vi "Draw Highlighted Tree rows.vi"(8 "error in (no error)":errorcluster, 9 "DragOver Output":T2={"Displayed Row"=0, "Position"=enum."On Row", "Row's TreeItem index"=0, "indent"=0, "Accepted?"=FALSE, "Insertion index"=0, "Top left visible TreeItem index"=0, "Bar type"=enum."tilda up"}, 10 "TreeItems":T1[](array[typedef]), 11 "TreeRef":refnum<vi>) -> (0 "error out":errorcluster)   [LabVIEW 2020, in "BetterDragAndDrop.lvlib" / "BetterTreeHandle.lvclass"]
uses:
  Classes/BetterTreeHandle/BetterTreeHandle.lvclass
  DragOver Output.ctl
  DragOverPosition.ctl
  Classes/BetterTreeBar/SubVIs/Horizontal Bar Enumeration.ctl
  Classes/BetterTreeItem/SubVIs/TreeItem.ctl
  Classes/BetterHandle/BetterHandle.lvclass
  Classes/BetterTreeBar/BetterHorizontalBar.lvclass
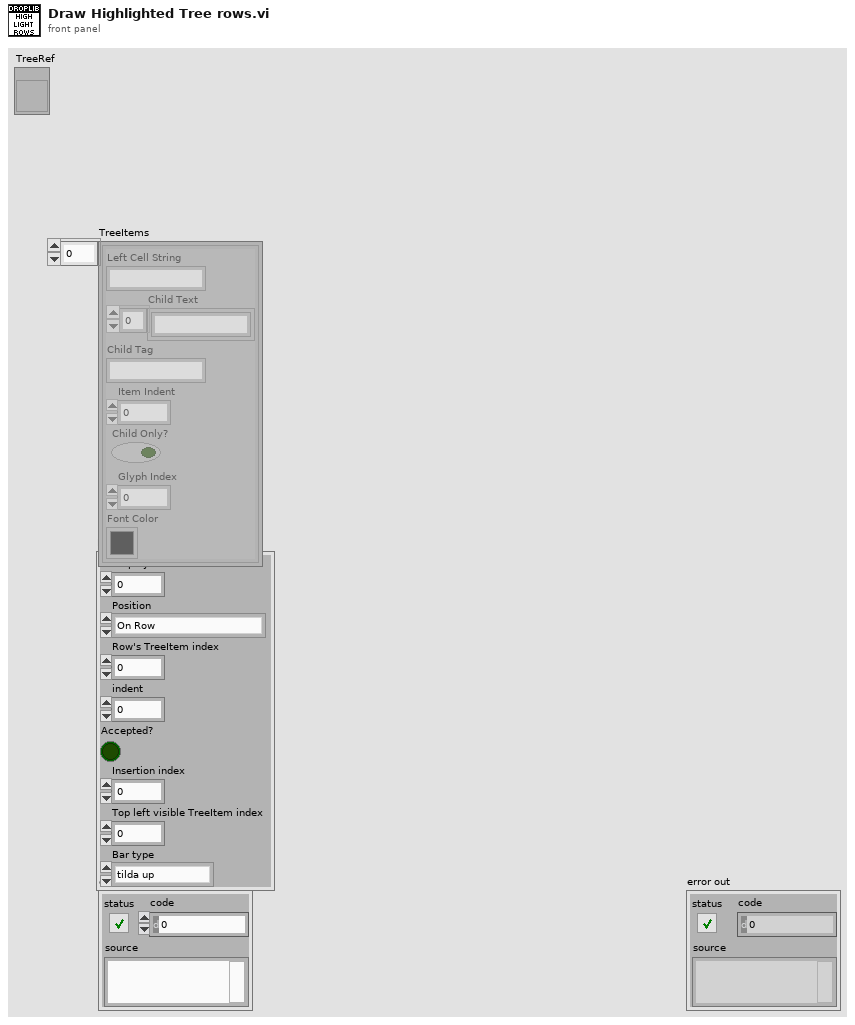
[diagram p1: front panel]
types:
  T1 = typedef "BetterDragAndDrop.lvlib/BetterTreeHandle.lvclass/TreeItem.ctl" = cluster{"Left Cell String":string, "Child Text":string[], "Child Tag":string, "Item Indent":i32, "Child Only?":bool, "Glyph Index":i32, "Font Color":u32}
  T2 = typedef "BetterDragAndDrop.lvlib/BetterHandle.lvclass/DragOver Output.ctl" = cluster{"Displayed Row":i32, "Position":T3, "Row's TreeItem index":i32, "indent":i32, "Accepted?":bool, "Insertion index":i32, "Top left visible TreeItem index":i32, "Bar type":T4}
  T3 = typedef "BetterDragAndDrop.lvlib/BetterHandle.lvclass/DragOverPosition.ctl" = enum16{"On Row", "Inbetween"}
  T4 = typedef "BetterDragAndDrop.lvlib/BetterHorizontalBar.lvclass/Horizontal Bar Enumeration.ctl" = enum16{"None", "only bar", "tilda up"}
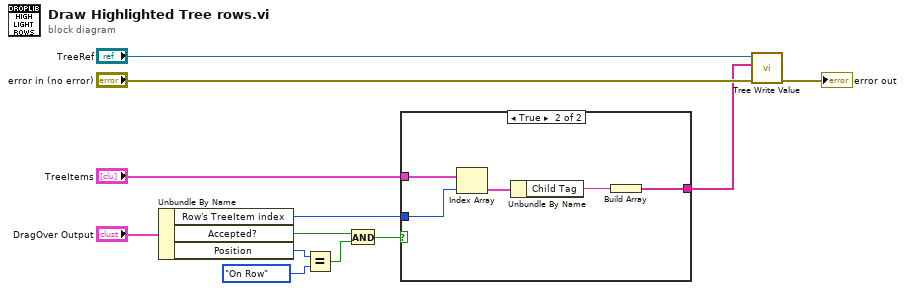
[diagram p0: block diagram]
diagram:
  n1 = Unbundle By Name("DragOver Output") -> ("Row's TreeItem index"=w11:i32, "Accepted?"=w7:bool, "Position"=w8:T3)
  n2 = Equal?(x=w8, y=DragOverPosition."On Row" ("Position")) -> (x = y?=w6:bool)
  n3 = And(x=w7, y=w6) -> (x .and. y?=w5:bool)
  n4 = case shown="True" w5 {
    tunnel: w11 -> [_ w16]
    tunnel: [_ w13] -> w1
    tunnel: "TreeItems" -> [_ w14]
    frame False {
    }
    frame True {
      n5 = Index Array(array=w14, index=w16) -> (element=w17:T1)
      n6 = Unbundle By Name(w17) -> ("Child Tag"=w15:string)
      n7 = Build Array(w15) -> (w13:string[])
    }
  }
  n8 = call "Tree Write Value.vi"("error in (no error)"="error in (no error)", "Value"=w1, "Tree Ref (generic)"="TreeRef") -> ("error out"=→"error out":errorcluster)  [unwired: 7 in, 1 out]
